vi "Image Process (Alex Angelillo's conflicted copy 2013-03-22).vi"(7 "Particle Measurements (Pixels)":dbl[][](array[numeric]) format="%.2f", 8 "Vision PID gains":T1={"proportional gain (Kc)"=0.2, "integral time (Ti, min)"=0.0, "derivative time (Td, min)"=0.0} {"derivative time (Td, min)" format="%.3f"; "integral time (Ti, min)" format="%.3f"; "proportional gain (Kc)" format="%.3f"}) -> (0 "Motor Output":dbl=0.96, 2 "String":string="0.960000")   [LabVIEW 2012]
uses:
  <vilib>/addons/control/pid/pid.llb/PID (DBL).vi
  <vilib>/addons/control/pid/NI_PID_pid.lvlib
panel:
  in  "Vision PID limits":cluster{"output high":dbl, "output low":dbl}={"output high"=1.0, "output low"=-1.0} {"output low" format="%.2f"; "output high" format="%.2f"}
  # "P= 0.003\nI = 0\nD = 0"
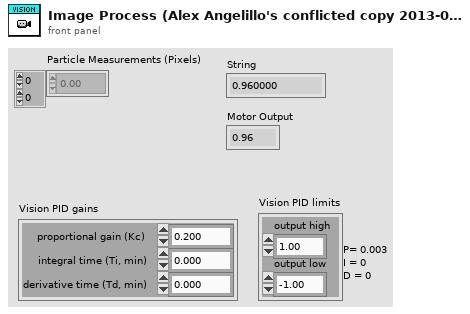
[diagram p1: front panel]
types:
  T1 = cluster{"proportional gain (Kc)":dbl, "integral time (Ti, min)":dbl, "derivative time (Td, min)":dbl}
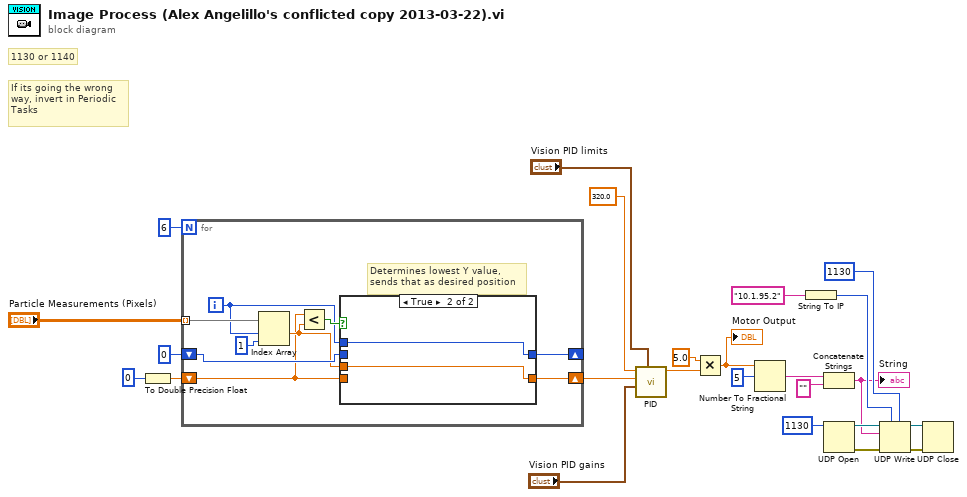
[diagram p0: block diagram]
diagram:
  # "If its going the wrong\nway, invert in Periodic\nTasks"
  # "1130 or 1140"
  n1 = To Double Precision Float(number=0) -> (double precision float=w12:dbl)
  n2 = for {
    N: 6 -> [_]
    tunnel: "Particle Measurements (Pixels)" -> [w32] mode=indexing
    shift-right: [w29] -> w11
    shift-left: w12 -> [w25]
    shift-right: [w28] -> _
    shift-left: 0 -> [w30]
    i -> [w31]
    # "Determines lowest Y value,\nsends that as desired position"
    n3 = Index Array(array=w32, index #1=w31, index #2=1 ("disabled index (col)")) -> (element #1=w26:dbl)  [unwired: 1 out]
    n4 = Less?(x=w25, y=w26) -> (x < y?=w33:bool)
    n5 = case shown="True" w33 {
      tunnel: w31 -> [_ w37]
      tunnel: [w34 w37] -> w28
      tunnel: w26 -> [_ w36]
      tunnel: [w35 w36] -> w29
      tunnel: w25 -> [w35 _]
      tunnel: w30 -> [w34 _]
      frame False {
      }
      frame True {
      }
    }
  }
  n6 = call-poly <vilib>:"PID.vi"("output range"="Vision PID limits", "PID gains"="Vision PID gains", "process variable"=w11, "setpoint"=320.0) -> ("output"=w3:dbl)  [unwired: 6 in, 1 out]
  n7 = Multiply(x=5.0, y=w3) -> (x*y=w2:dbl)
  "Motor Output" <- w2
  n8 = Number To Fractional String(number=w2, width (-)=i16 5) -> (F-format string=w5:string)  [unwired: 2 in]
  n9 = String To IP(1:"10.1.95.2" ("name")) -> (0:w18:u32)
  n10 = Concatenate Strings(w5, "" ("string")) -> (w7:string)
  "String" <- w7
  n11 = UDP Open(11:u16 1130 ("port")) -> (port=w23:refnum<k16>, 0:w22:errorcluster)  [unwired: 4 in, 1 out]
  n12 = UDP Write(address=w18, port or service name=u16 1130, connection ID=w23, data in=w7, 8:w22) -> (error out=w21:errorcluster, 3:w20:refnum<k16>)  [unwired: 1 in]
  n13 = UDP Close(connection ID=w20, 8:w21) -> ()  [unwired: 2 out]
